vi "GenericEdge.vi"() -> ()   [LabVIEW 2015]
panel:
  out "Properties from ThingWorx":string[][](array[string])=[["Button", "false"], ["Button2", "false"], ["description", ""], ["isConnected", "false"], ["lastConnection", "1970-01-01T00:00:00.000Z"], ["name", "GenericEdge"], ["Photocell", "200.0"], ["Potentiometer", "234.0"], ["tags", "GenericRemoteEdge:Example"], ["Temperature", "2.42"], ["thingTemplate", "GenericThingTemplate"]]
  in  "End Session":bool
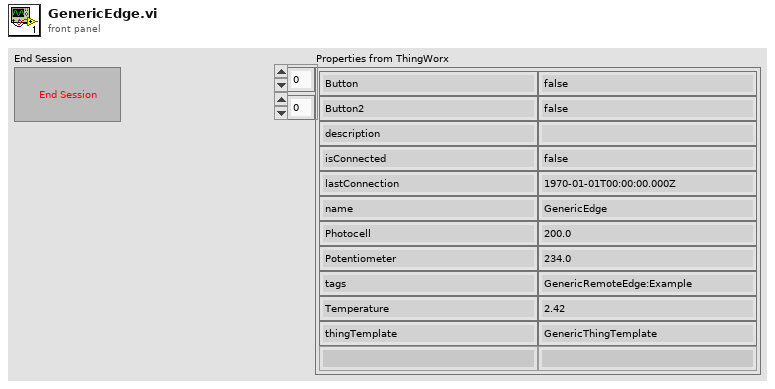
[diagram p1: front panel]
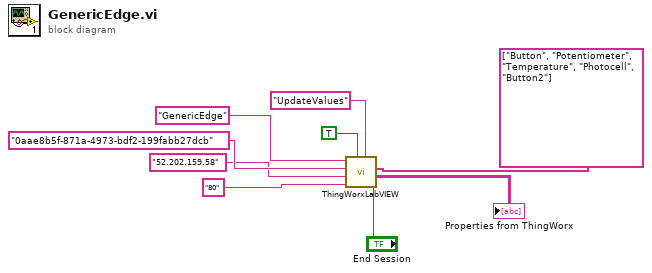
[diagram p0: block diagram]
diagram:
  n1 = call "ThingWorxLabVIEW.vi"("End Session"="End Session", "Properties in Service"=string[] ["Button", "Potentiometer", "Temperature", "Photocell", "Button2"], "Service Name"="UpdateValues", "Continuous?"=TRUE, "Port"="80", "ThingWorx Server Address"="52.202.159.58", "App Key"="0aae8b5f-871a-4973-bdf2-199fabb27dcb", "Thing Name"="GenericEdge") -> ("Properties from ThingWorx"=→"Properties from ThingWorx":string[][])  [unwired: 3 in]
